vi "Format.vi"(5 "Force Safe Mode (F)":bool, 6 "Timeout (90,000 ms)":u32=90000, 7 "Restart After Format (T)":bool=TRUE, 8 "error in (no error)":errorcluster, 9 "Keep Network Settings (F)":bool, 10 "File System":T1 items=["Default"=0, "FAT"=1, "Reliance"=2, "UBIFS"=16384, "Ext4"=32768], 11 "Session in":refnum<k21>) -> (0 "error out":errorcluster, 3 "Session out":refnum<k21>)   [LabVIEW 2014, in "nisyscfg.lvlib"]
doc: "Erases all data from the primary hard drive of a system. If the system is not in user-directed safe mode and <B>force safe mode</B> is FALSE, this VI will return an error."
uses:
  nisyscfg.lvlib
  File System.ctl
  Network Settings Format.ctl
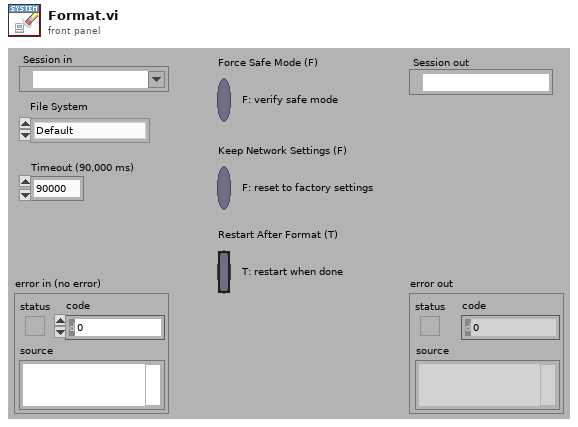
[diagram p1: front panel]
types:
  T1 = typedef "nisyscfg.lvlib/File System.ctl" = i32
  T2 = typedef "nisyscfg.lvlib/Network Settings Format.ctl" = u32
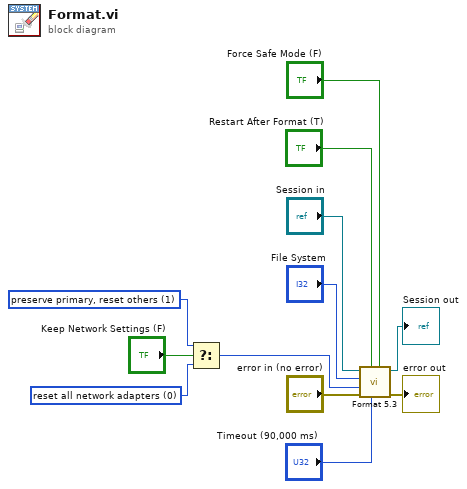
[diagram p0: block diagram]
diagram:
  w11 = T2 1 items=["reset all network adapters", "preserve primary, reset others", "preserve all network adapters"] ("network settings (reset all adapters)")
  w10 = T2 0 items=["reset all network adapters", "preserve primary, reset others", "preserve all network adapters"] ("network settings (reset all adapters)")
  n1 = Select(t=w11, s="Keep Network Settings (F)", f=w10) -> (s? t:f=w4:T2)
  n2 = call "Format 5.3.vi"("Force Safe Mode (F)"="Force Safe Mode (F)", "Timeout (300,000 ms)"="Timeout (90,000 ms)", "Restart After Format (T)"="Restart After Format (T)", "error in (no error)"="error in (no error)", "Network Settings (reset all adapters)"=w4, "File System"="File System", "Session in"="Session in") -> ("error out"=→"error out":errorcluster, "Session out"=→"Session out":refnum<k21>)  [unwired: 3 in]
